vi "Log View for Cross Spectrum.vi"(2 "channel Y info":T1={"sensor sensitivity [mV/EU]"=1000.0, "engineering units"=1, "dB reference [EU]"=1.0, "custom label"="EU", "weighting filter"=0, "pregain [dB]"=0.0} {"pregain [dB]" format="%.2f"; "weighting filter" items=["Linear", "A-weighting", "B-weighting", "C-weighting", "ITU-R 468-4", "Dolby", "CCITT", "C-message"]; "dB reference [EU]" format="%^.1e"; "engineering units" items=["custom..."=0, "V"=1, "A"=21, "Pa"=2, "N"=20, "g"=3, "m/s^2"=4, "m/s"=5, "m"=6, "mm/s"=12, "mm"=13, "microns/s"=14, "microns"=15, "in/s^2"=7, "in/s"=8, "in"=9, "mils/s"=10, "mils"=11, "rad/s^2"=16, "rad/s"=17, "rad"=18, "strain"=19]; "sensor sensitivity [mV/EU]" format="%.2f"}, 3 "channel X info":T1={"sensor sensitivity [mV/EU]"=1000.0, "engineering units"=1, "dB reference [EU]"=1.0, "custom label"="EU", "weighting filter"=0, "pregain [dB]"=0.0} {"pregain [dB]" format="%.2f"; "weighting filter" items=["Linear", "A-weighting", "B-weighting", "C-weighting", "ITU-R 468-4", "Dolby", "CCITT", "C-message"]; "dB reference [EU]" format="%^.1e"; "engineering units" items=["custom..."=0, "V"=1, "A"=21, "Pa"=2, "N"=20, "g"=3, "m/s^2"=4, "m/s"=5, "m"=6, "mm/s"=12, "mm"=13, "microns/s"=14, "microns"=15, "in/s^2"=7, "in/s"=8, "in"=9, "mils/s"=10, "mils"=11, "rad/s^2"=16, "rad/s"=17, "rad"=18, "strain"=19]; "sensor sensitivity [mV/EU]" format="%.2f"}, 4 "dB On (T)":bool=TRUE, 5 "cross spectrum [EUx EUy rms]":dbl[](array[numeric]) format="%.2f") -> (0 "unit label":string, 1 "log view cross spectrum [dB EUx EUy]":dbl[](array[numeric]) format="%.2f")   [LabVIEW 2017]
uses:
  <vilib>/addons/Sound and Vibration/compatibility/Controls/svl_Channel Info.ctl
  <vilib>/addons/Sound and Vibration/compatibility/Controls/svl_Engineering Units Text Ring.ctl
  <vilib>/addons/Sound and Vibration/compatibility/Controls/svl_Weighting Filter Text Ring.ctl
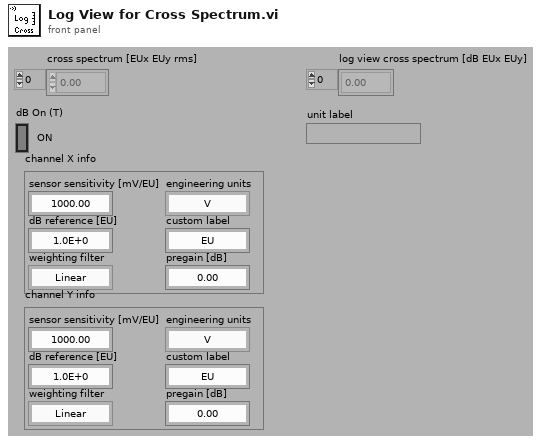
[diagram p1: front panel]
types:
  T1 = typedef "svl_Channel Info.ctl" = cluster{"sensor sensitivity [mV/EU]":dbl, "engineering units":T2, "dB reference [EU]":dbl, "custom label":string, "weighting filter":T3, "pregain [dB]":dbl}
  T2 = typedef "svl_Engineering Units Text Ring.ctl" = u16
  T3 = typedef "svl_Weighting Filter Text Ring.ctl" = u16
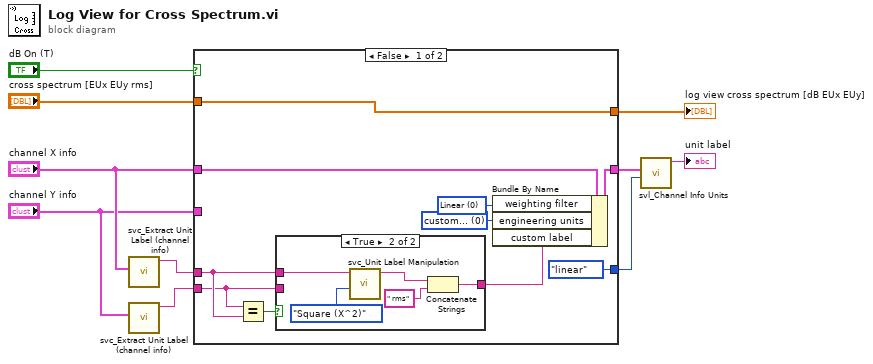
[diagram p0: block diagram]
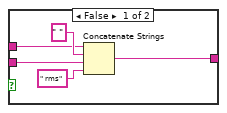
[diagram p2: hidden frame]
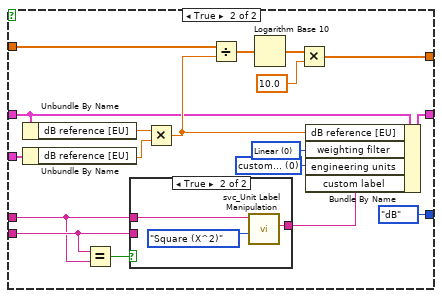
[diagram p3: hidden frame]
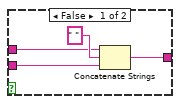
[diagram p4: hidden frame]
diagram:
  n1 = call <vilib>:"svc_Extract Unit Label (channel info).vi"("channel info"="channel X info") -> ("unit label"=w4:string)  [unwired: 8 in, 2 out]
  n2 = call <vilib>:"svc_Extract Unit Label (channel info).vi"("channel info"="channel Y info") -> ("unit label"=w5:string)  [unwired: 8 in, 2 out]
  n3 = case shown="False" "dB On (T)" {
    tunnel: [w17 w44] -> w8
    tunnel: "cross spectrum [EUx EUy rms]" -> [w17 w45]
    tunnel: w4 -> [w19 w38]
    tunnel: w5 -> [w18 w39]
    tunnel: "channel X info" -> [w16 w33]
    tunnel: "channel Y info" -> [_ w43]
    tunnel: [w15 w34] -> w3
    tunnel: [enum16{"linear", "dB"}."linear" ("linear/dB") enum16{"linear", "dB"}."dB" ("linear/dB")] -> w1
    frame False {
      w12 = u16 0 items=["Linear", "A-weighting", "B-weighting", "C-weighting"] ("weighting filter")
      w13 = u16 0 items=["custom...", "V", "Pa", "g", "m/s^2", "m/s", "m", "in/s^2", "in/s", "in", "mm", "mils", "A"] ("engineering units")
      n4 = Equal?(x=w18, y=w19) -> (x = y?=w20:bool)
      n5 = case shown="True" w20 {
        tunnel: [w21 w26] -> w14
        tunnel: w19 -> [w24 w27]
        tunnel: w18 -> [w23 _]
        frame False {
          n6 = Concatenate Strings(w24, " " ("custom label"), w23, " rms") -> (w21:string)
        }
        frame True {
          n7 = call <vilib>:"svc_Unit Label Manipulation.vi"("operation"=enum16{"Square (X^2)", "Divide (X/Y)"}."Square (X^2)", "X unit label"=w27) -> ("resulting unit label"=w29:string)  [unwired: 5 in]
          n8 = Concatenate Strings(w29, " rms") -> (w26:string)
        }
      }
      n9 = Bundle By Name(cluster=w16, "weighting filter"=w12, "engineering units"=w13, "custom label"=w14) -> (w15:T1)
    }
    frame True {
      w31 = T2 0 items=["custom..."=0, "V"=1, "A"=21, "Pa"=2, "N"=20, "g"=3, "m/s^2"=4, "m/s"=5, "m"=6, "mm/s"=12, "mm"=13, "microns/s"=14, "microns"=15, "in/s^2"=7, "in/s"=8, "in"=9, "mils/s"=10, "mils"=11, "rad/s^2"=16, "rad/s"=17, "rad"=18, "strain"=19] ("engineering units")
      w32 = T3 0 items=["Linear", "A-weighting", "B-weighting", "C-weighting", "ITU-R 468-4", "Dolby", "CCITT", "C-message"] ("weighting filter")
      n10 = Unbundle By Name(w33) -> ("dB reference [EU]"=w42:dbl)
      n11 = Unbundle By Name(w43) -> ("dB reference [EU]"=w41:dbl)
      n12 = Equal?(x=w39, y=w38) -> (x = y?=w40:bool)
      n13 = case shown="True" w40 {
        tunnel: w38 -> [w51 w55]
        tunnel: w39 -> [w50 _]
        tunnel: [w49 w54] -> w36
        frame False {
          n14 = Concatenate Strings(w51, " " ("custom label"), w50) -> (w49:string)
        }
        frame True {
          n15 = call <vilib>:"svc_Unit Label Manipulation.vi"("operation"=enum16{"Square (X^2)", "Divide (X/Y)"}."Square (X^2)", "X unit label"=w55) -> ("resulting unit label"=w54:string)  [unwired: 5 in]
        }
      }
      n16 = Multiply(x=w42, y=w41) -> (x*y=w35:dbl)
      n17 = Divide(x=w45, y=w35) -> (x/y=w48:dbl[])
      n18 = Logarithm Base 10(1:w48) -> (0:w46:dbl[])
      n19 = Multiply(x=w46, y=10.0) -> (x*y=w44:dbl[])
      n20 = Bundle By Name(cluster=w33, "dB reference [EU]"=w35, "weighting filter"=w32, "engineering units"=w31, "custom label"=w36) -> (w34:T1)
    }
  }
  "log view cross spectrum [dB EUx EUy]" <- w8
  n21 = call <vilib>:"svl_Channel Info Units.vi"("linear/dB"=w1, "channel info"=w3) -> ("unit label"=→"unit label":string)  [unwired: 8 in, 1 out]
